vi "Treatment.vi"(8 "error in (no error)":errorcluster caption="entrée d'erreur (pas d'erreur)", 11 "Load_Digits en entrée":refnum<class "Load_Digits.lvclass">) -> (0 "error out":errorcluster caption="sortie d'erreur", 2 "String 3DArray":cluster{"Data":string[][]}[](array[cluster]), 3 "Load_Digits en sortie":refnum<class "Load_Digits.lvclass">)   [LabVIEW 2020, in "Load_Digits.lvclass"]
uses:
  Load_Digits.lvclass
  Load_Digits.lvclass/Load_Digits.ctl
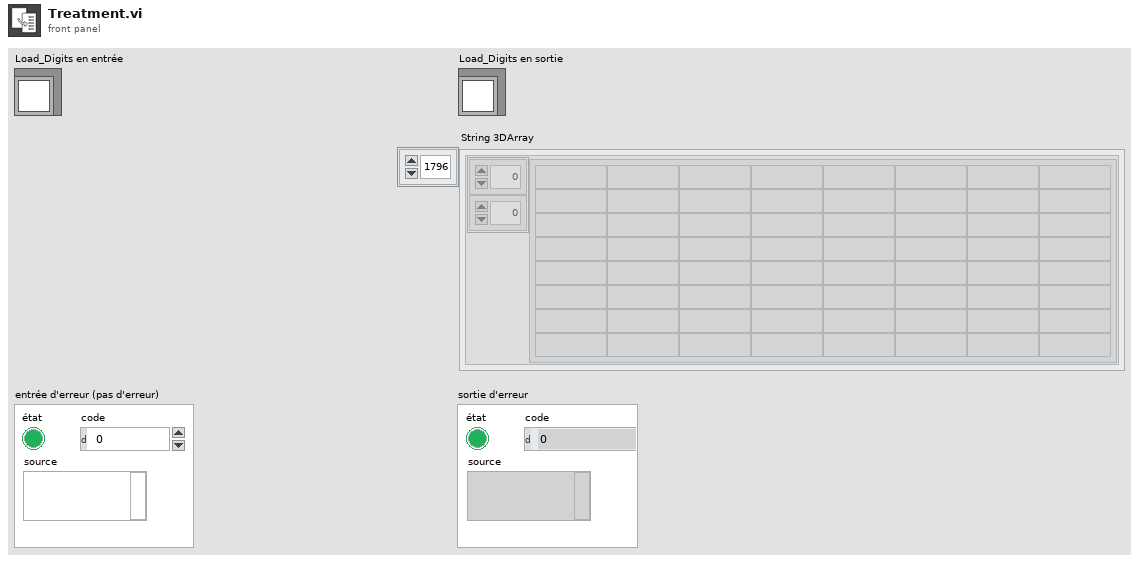
[diagram p1: front panel]
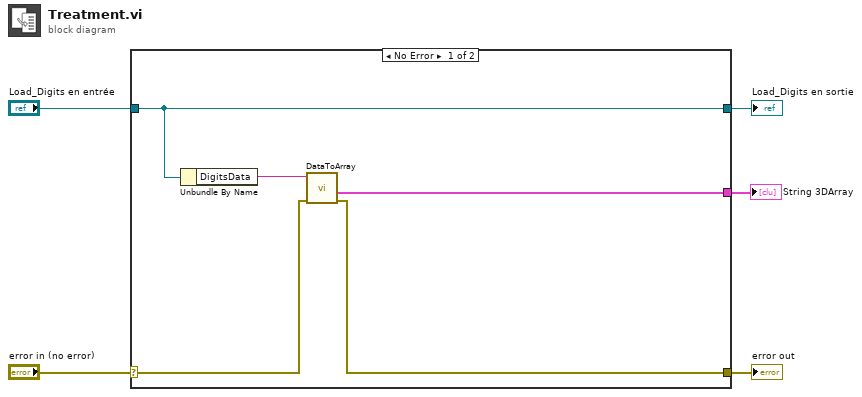
[diagram p0: block diagram]
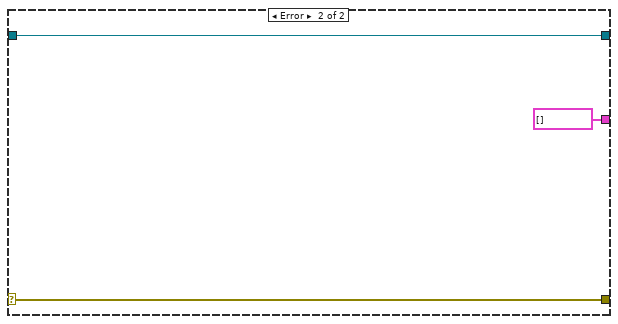
[diagram p2: hidden frame]
diagram:
  n1 = case shown="No Error" "error in (no error)" {
    selector: "error in (no error)" -> [w8 w13]
    tunnel: [w7 w13] -> w4
    tunnel: [w10 w12] -> w2
    tunnel: "Load_Digits en entrée" -> [w10 w12]
    tunnel: [w6 cluster{"Tableau":string[][]}[] [] ("String 3DArray")] -> w1
    frame No Error {
      n2 = Unbundle By Name(w10) -> ("DigitsData"=w9:string)
      n3 = call "DataToArray.vi"("sortie d'erreur"=w8, "Return value"=w9) -> ("sortie d'erreur"=w7:errorcluster, "String 3DArray"=w6:cluster{"Tableau":string[][]}[])  [unwired: 6 in, 2 out]
    }
    frame Error {
    }
  }
  "error out" <- w4
  "Load_Digits en sortie" <- w2
  "String 3DArray" <- w1
